vi "Find Scrubber For Date.vi"(8 "error in":errorcluster, 10 "Sample Date":string) -> (0 "error out":errorcluster, 2 "Found?":bool, 3 "Date Scrubber out":refnum<class "Date Scrubber.lvclass">)   [LabVIEW 2020, in "Approval Tests.lvlib" / "Date Scrubber.lvclass"]
uses:
  Date Scrubber.lvclass
  Regex Scrubber Count Unique/Regex Scrubber Count Unique.lvclass
  Regex Scrubber Count Unique/Regex Scrubber Count Unique.lvclass/Regex Scrubber Count Unique.ctl
  Date Scrubber.lvclass/Date Scrubber.ctl
  Regex Scrubber Count Unique/Write Prefix.vi
  Regex Scrubber Count Unique/Write Regex.vi
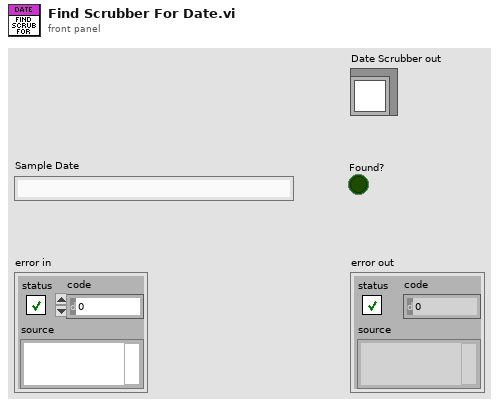
[diagram p1: front panel]
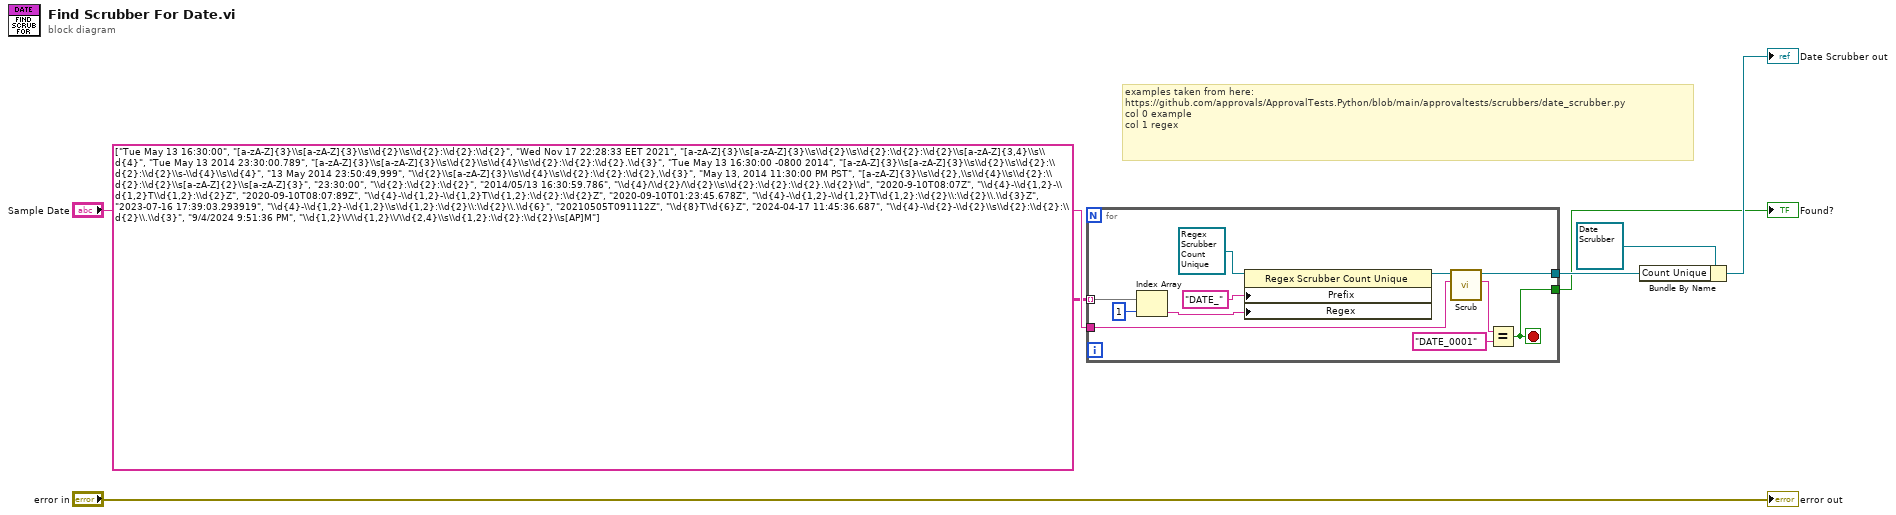
[diagram p0: block diagram]
diagram:
  # "examples taken from here:\nhttps://github.com/approvals/ApprovalTests.Python/blob/main/approvaltests/scrubbers/date_scrubber.py\ncol 0 example\ncol 1 regex"
  n1 = for {
    tunnel: [w12] -> w4
    tunnel: string[][] [["Tue May 13 16:30:00", "[a-zA-Z]{3}\\s[a-zA-Z]{3}\\s\\d{2}\\s\\d{2}:\\d{2}:\\d{2}"], ["Wed Nov 17 22:28:33 EET 2021", "[a-zA-Z]{3}\\s[a-zA-Z]{3}\\s\\d{2}\\s\\d{2}:\\d{2}:\\d{2}\\s[a-zA-Z]{3,4}\\s\\d{4}"], ["Tue May 13 2014 23:30:00.789", "[a-zA-Z]{3}\\s[a-zA-Z]{3}\\s\\d{2}\\s\\d{4}\\s\\d{2}:\\d{2}:\\d{2}.\\d{3}"], ["Tue May 13 16:30:00 -0800 2014", "[a-zA-Z]{3}\\s[a-zA-Z]{3}\\s\\d{2}\\s\\d{2}:\\d{2}:\\d{2}\\s-\\d{4}\\s\\d{4}"], ["13 May 2014 23:50:49,999", "\\d{2}\\s[a-zA-Z]{3}\\s\\d{4}\\s\\d{2}:\\d{2}:\\d{2},\\d{3}"], ["May 13, 2014 11:30:00 PM PST", "[a-zA-Z]{3}\\s\\d{2},\\s\\d{4}\\s\\d{2}:\\d{2}:\\d{2}\\s[a-zA-Z]{2}\\s[a-zA-Z]{3}"], ["23:30:00", "\\d{2}:\\d{2}:\\d{2}"], ["2014/05/13 16:30:59.786", "\\d{4}/\\d{2}/\\d{2}\\s\\d{2}:\\d{2}:\\d{2}.\\d{2}\\d"], ["2020-9-10T08:07Z", "\\d{4}-\\d{1,2}-\\d{1,2}T\\d{1,2}:\\d{2}Z"], ["2020-09-10T08:07:89Z", "\\d{4}-\\d{1,2}-\\d{1,2}T\\d{1,2}:\\d{2}:\\d{2}Z"], ["2020-09-10T01:23:45.678Z", "\\d{4}-\\d{1,2}-\\d{1,2}T\\d{1,2}:\\d{2}\\:\\d{2}\\.\\d{3}Z"], ["2023-07-16 17:39:03.293919", "\\d{4}-\\d{1,2}-\\d{1,2}\\s\\d{1,2}:\\d{2}\\:\\d{2}\\.\\d{6}"], ["20210505T091112Z", "\\d{8}T\\d{6}Z"], ["2024-04-17 11:45:36.687", "\\d{4}-\\d{2}-\\d{2}\\s\\d{2}:\\d{2}:\\d{2}\\.\\d{3}"], ["9/4/2024 9:51:36 PM", "\\d{1,2}\\/\\d{1,2}\\/\\d{2,4}\\s\\d{1,2}:\\d{2}:\\d{2}\\s[AP]M"]] -> [w16] mode=indexing
    tunnel: "Sample Date" -> [w11]
    tunnel: [w8] -> w2
    stop <- w8 stop-if-true
    n2 = Index Array(array=w16, index=1) -> (element=w14:string)
    n3 = property class="Regex Scrubber Count Unique"(reference=refnum<class "Regex Scrubber Count Unique.lvclass"> refnum ("Approval Tests.lvlib:Regex Scrubber Count Unique"), "Prefix"="DATE_", "Regex"=w14) -> (reference out=w13:refnum<class "Regex Scrubber Count Unique.lvclass">)  [unwired: 1 in, 1 out]
    n4 = call-dynamic "Scrub.vi"("Input String"=w11, "Regex Scrubber in"=w13) -> ("Scrubbed String"=w10:string, "Regex Scrubber out"=w12:refnum<class "Regex Scrubber Count Unique.lvclass">)  [unwired: 7 in, 1 out]
    n5 = Equal?(x=w10, y="DATE_0001") -> (x = y?=w8:bool)
  }
  "Found?" <- w2
  n6 = Bundle By Name(cluster=refnum<class "Date Scrubber.lvclass"> refnum ("Date Scrubber out"), "Count Unique"=w4) -> (→"Date Scrubber out":refnum<class "Date Scrubber.lvclass">)
  "error out" <- "error in"
